vi "Red Pitaya Test.vi"(8 "Error In":errorcluster, 10 "Server port":u16=1002, 11 "Server address":string="192.168.1.100") -> (0 "Error Out":errorcluster)   [LabVIEW 2024]
uses:
  RP Command.ctl
  RP EEPROM Calibration.ctl
  RP Calibration.ctl
  RP Calibration 4ch.ctl
  RP Channel Calibration.ctl
  RP Filter 4ch.ctl
  RP Channel Filter.ctl
  RP Calibration 2ch.ctl
  RP Write Command TCP.vi
panel:
  out "Armed":bool
  in  "Trigger":bool
  in  "Arm":bool
  out "Numeric":dbl
  in  "length (rest)":i32
  in  "offset (0)":i32
  out "CH Calibration length":i32
  out "RP Calibration length":i32
  in  "New calibration format":bool=TRUE
  out "RP Calibration":T1
  out "RP EEPROM Calibration":T7 {"magic" format="%x"}
  in  "New connection":bool
  out "data out":string
  in  "Command payload":u64 format="%x"
  in  "Send Button":bool
  in  "Process Stop Button":bool
  in  "Command number":T8
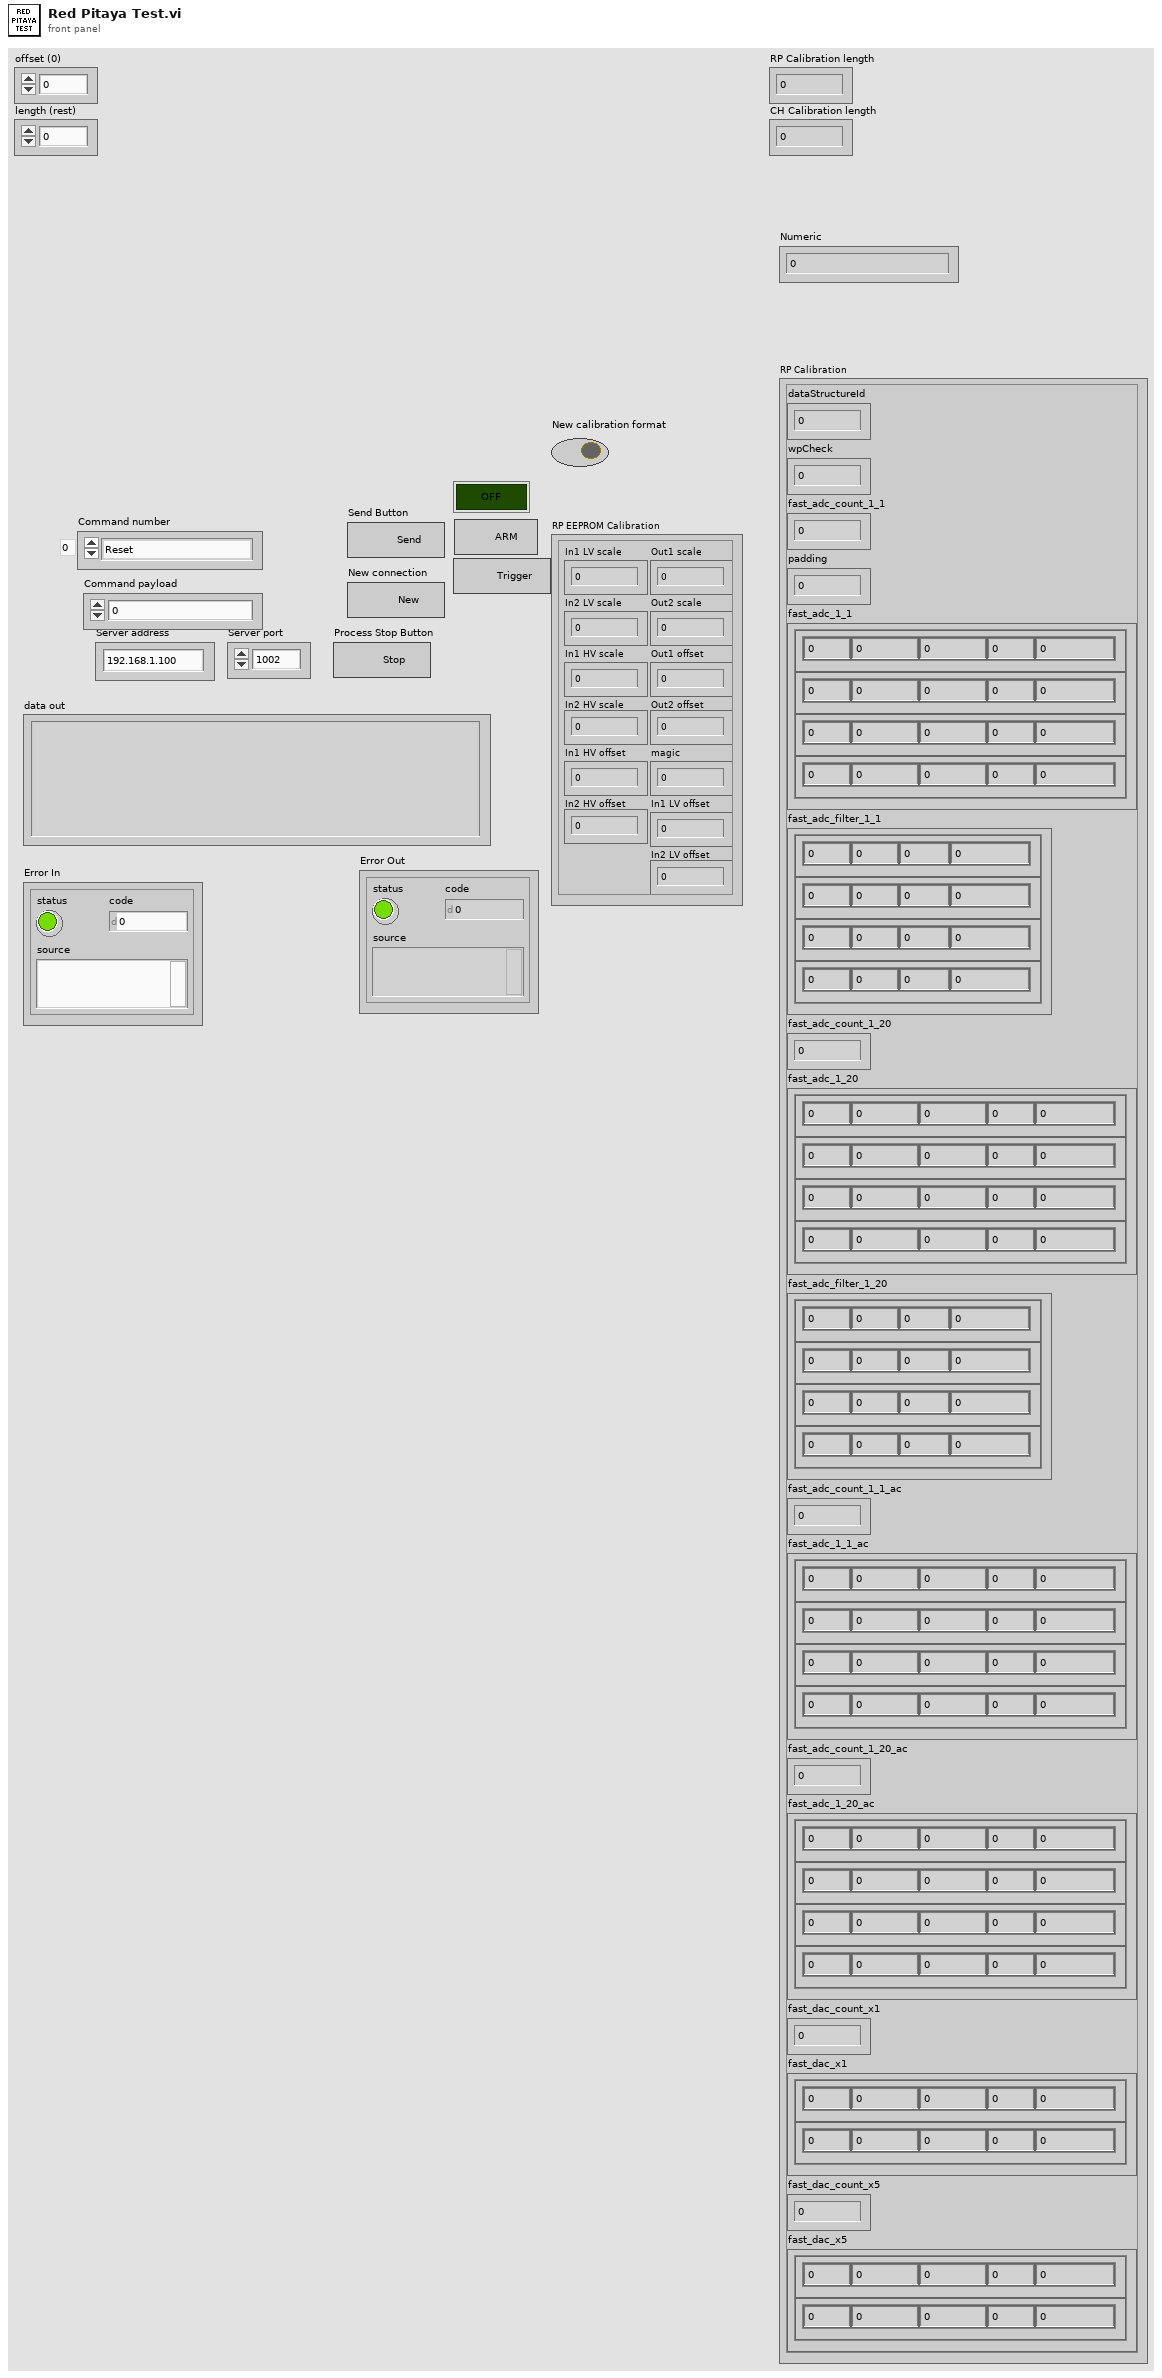
[diagram p1: front panel]
types:
  T1 = typedef "RP Calibration.ctl" = cluster{"dataStructureId":u8, "wpCheck":u8, "fast_adc_count_1_1":u16, "padding":u32, "fast_adc_1_1":T2, "fast_adc_filter_1_1":T4, "fast_adc_count_1_20":u64, "fast_adc_1_20":T2, "fast_adc_filter_1_20":T4, "fast_adc_count_1_1_ac":u64, "fast_adc_1_1_ac":T2, "fast_adc_count_1_20_ac":u64, "fast_adc_1_20_ac":T2, "fast_dac_count_x1":u64, "fast_dac_x1":T6, "fast_dac_count_x5":u64, "fast_dac_x5":T6}
  T2 = typedef "RP Calibration 4ch.ctl" = cluster{"ch_0":T3, "ch_1":T3, "ch_2":T3, "ch_3":T3}
  T3 = typedef "RP Channel Calibration.ctl" = cluster{"baseScale":sgl, "calibValue":u32, "offset":i32, "padding 2":i32, "gainCalc":dbl}
  T4 = typedef "RP Filter 4ch.ctl" = cluster{"ch_0":T5, "ch_1":T5, "ch_2":T5, "ch_3":T5}
  T5 = typedef "RP Channel Filter.ctl" = cluster{"aa":u32, "bb":u32, "pp":u32, "kk":u32}
  T6 = typedef "RP Calibration 2ch.ctl" = cluster{"ch_0":T3, "ch_1":T3}
  T7 = typedef "RP EEPROM Calibration.ctl" = cluster{"In1 LV scale":u32, "In2 LV scale":u32, "In1 HV scale":u32, "In2 HV scale":u32, "In1 HV offset":i32, "In2 HV offset":i32, "Out1 scale":u32, "Out2 scale":u32, "Out1 offset":i32, "Out2 offset":i32, "magic":u32, "In1 LV offset":i32, "In2 LV offset":i32}
  T8 = typedef "RP Command.ctl" = enum16{"Reset", "Read IDN", "Stop server", "Get status", "Get temperature", "Connect client", "Arm", "Software trigger", "Get whole buffer", "Get chunk", "System call", "Get config", "Set config", "Recieve data", "Recieve Calibartion", "Transmit data"}
  T9 = enum16{"big-endian, network order", "native, host order", "little-endian"}
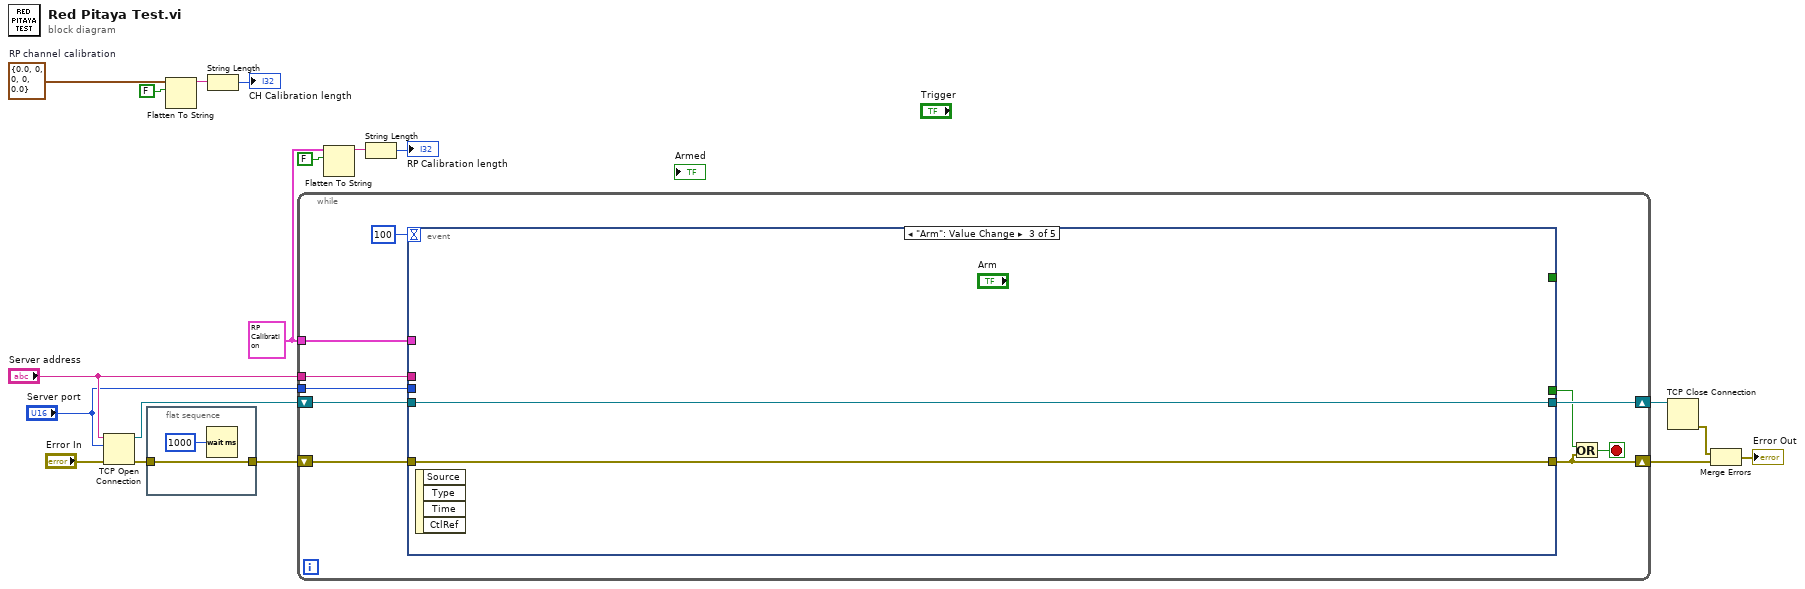
[diagram p0: block diagram]
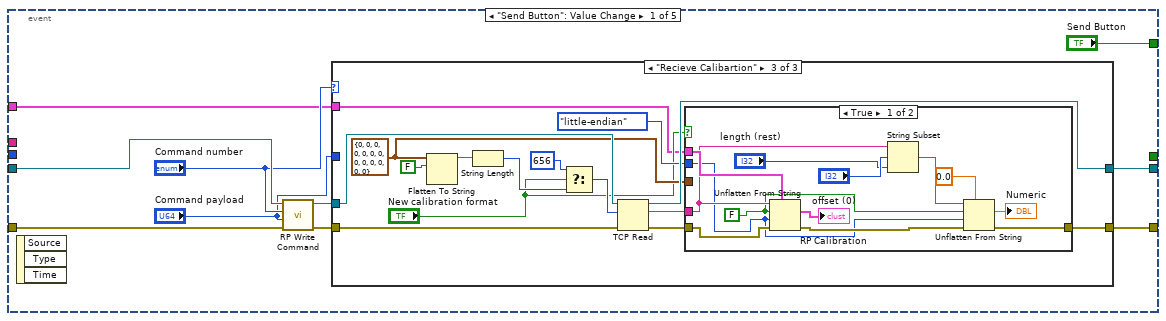
[diagram p2: hidden frame]
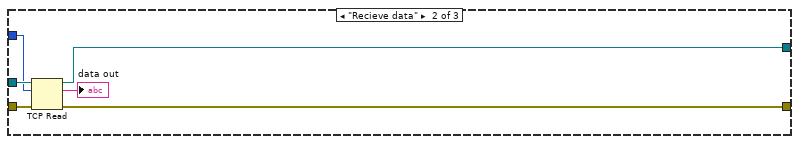
[diagram p4: hidden frame]
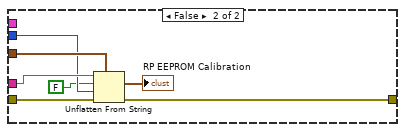
[diagram p5: hidden frame]
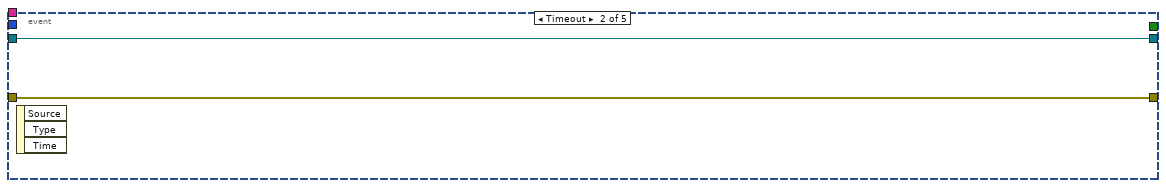
[diagram p6: hidden frame]
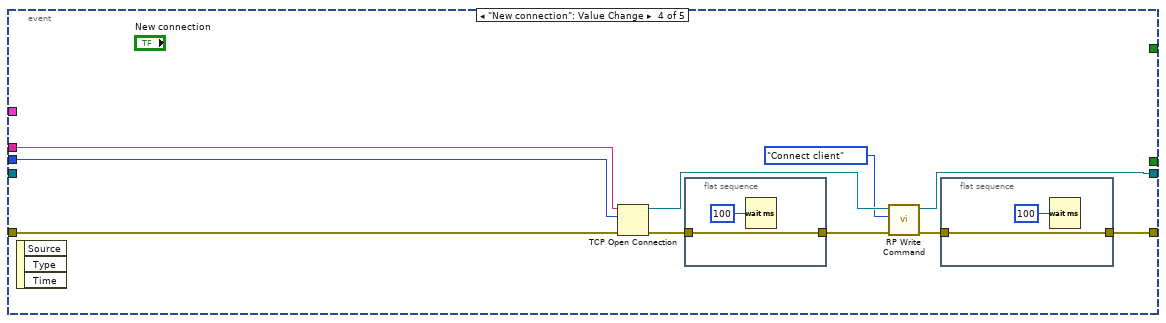
[diagram p7: hidden frame]
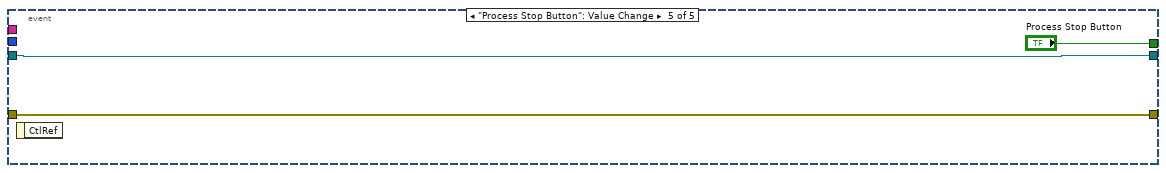
[diagram p8: hidden frame]
diagram:
  w1 = T1 {"dataStructureId"=0, "wpCheck"=0, "fast_adc_count_1_1"=0, "padding"=0, "fast_adc_1_1"={"ch_0"={"baseScale"=0.0, "calibValue"=0, "offset"=0, "padding 2"=0, "gainCalc"=0.0}, "ch_1"={"baseScale"=0.0, "calibValue"=0, "offset"=0, "padding 2"=0, "gainCalc"=0.0}, "ch_2"={"baseScale"=0.0, "calibValue"=0, "offset"=0, "padding 2"=0, "gainCalc"=0.0}, "ch_3"={"baseScale"=0.0, "calibValue"=0, "offset"=0, "padding 2"=0, "gainCalc"=0.0}}, "fast_adc_filter_1_1"={"ch_0"={"aa"=0, "bb"=0, "pp"=0, "kk"=0}, "ch_1"={"aa"=0, "bb"=0, "pp"=0, "kk"=0}, "ch_2"={"aa"=0, "bb"=0, "pp"=0, "kk"=0}, "ch_3"={"aa"=0, "bb"=0, "pp"=0, "kk"=0}}, "fast_adc_count_1_20"=0, "fast_adc_1_20"={"ch_0"={"baseScale"=0.0, "calibValue"=0, "offset"=0, "padding 2"=0, "gainCalc"=0.0}, "ch_1"={"baseScale"=0.0, "calibValue"=0, "offset"=0, "padding 2"=0, "gainCalc"=0.0}, "ch_2"={"baseScale"=0.0, "calibValue"=0, "offset"=0, "padding 2"=0, "gainCalc"=0.0}, "ch_3"={"baseScale"=0.0, "calibValue"=0, "offset"=0, "padding 2"=0, "gainCalc"=0.0}}, "fast_adc_filter_1_20"={"ch_0"={"aa"=0, "bb"=0, "pp"=0, "kk"=0}, "ch_1"={"aa"=0, "bb"=0, "pp"=0, "kk"=0}, "ch_2"={"aa"=0, "bb"=0, "pp"=0, "kk"=0}, "ch_3"={"aa"=0, "bb"=0, "pp"=0, "kk"=0}}, "fast_adc_count_1_1_ac"=0, "fast_adc_1_1_ac"={"ch_0"={"baseScale"=0.0, "calibValue"=0, "offset"=0, "padding 2"=0, "gainCalc"=0.0}, "ch_1"={"baseScale"=0.0, "calibValue"=0, "offset"=0, "padding 2"=0, "gainCalc"=0.0}, "ch_2"={"baseScale"=0.0, "calibValue"=0, "offset"=0, "padding 2"=0, "gainCalc"=0.0}, "ch_3"={"baseScale"=0.0, "calibValue"=0, "offset"=0, "padding 2"=0, "gainCalc"=0.0}}, "fast_adc_count_1_20_ac"=0, "fast_adc_1_20_ac"={"ch_0"={"baseScale"=0.0, "calibValue"=0, "offset"=0, "padding 2"=0, "gainCalc"=0.0}, "ch_1"={"baseScale"=0.0, "calibValue"=0, "offset"=0, "padding 2"=0, "gainCalc"=0.0}, "ch_2"={"baseScale"=0.0, "calibValue"=0, "offset"=0, "padding 2"=0, "gainCalc"=0.0}, "ch_3"={"baseScale"=0.0, "calibValue"=0, "offset"=0, "padding 2"=0, "gainCalc"=0.0}}, "fast_dac_count_x1"=0, "fast_dac_x1"={"ch_0"={"baseScale"=0.0, "calibValue"=0, "offset"=0, "padding 2"=0, "gainCalc"=0.0}, "ch_1"={"baseScale"=0.0, "calibValue"=0, "offset"=0, "padding 2"=0, "gainCalc"=0.0}}, "fast_dac_count_x5"=0, "fast_dac_x5"={"ch_0"={"baseScale"=0.0, "calibValue"=0, "offset"=0, "padding 2"=0, "gainCalc"=0.0}, "ch_1"={"baseScale"=0.0, "calibValue"=0, "offset"=0, "padding 2"=0, "gainCalc"=0.0}}} ("RP Calibration")
  w4 = T3 {"baseScale"=0.0, "calibValue"=0, "offset"=0, "padding 2"=0, "gainCalc"=0.0}  # RP channel calibration
  n1 = TCP Open Connection(address="Server address", remote port or service name="Server port", error in (no error)="Error In") -> (connection ID=w14:refnum<k5>, error out=w13:errorcluster)  [unwired: 2 in]
  n2 = flat-sequence {
    tunnel: w13 -> [w19]
    tunnel: [w19] -> w12
    frame #0 {
      n3 = Wait (ms)(milliseconds to wait=u32 1000) -> ()  [unwired: 1 out]
    }
  }
  n4 = Flatten To String(anything=w4, prepend array or string size? (T)=FALSE) -> (data string=w2:string)  [unwired: 2 in, 2 out]
  n5 = String Length(string=w2) -> (length=→"CH Calibration length":i32)
  n6 = while {
    shift-right: [w30] -> w16
    shift-left: w14 -> [w29]
    shift-right: [w25] -> w15
    shift-left: w12 -> [w28]
    tunnel: "Server address" -> [w23]
    tunnel: "Server port" -> [w22]
    tunnel: w1 -> [w21]
    stop <- w26 stop-if-true
    n7 = event shown="[2] \"Arm\": Value Change" {
      selector: _ -> [_ _ _ _ _]
      dyn-events: _ -> [_ _ _ _ _]
      timeout: 100 -> [_ _ _ _ _]
      tunnel: [w33 w85 w86 w88 w102] -> w30
      tunnel: [w32 w84 w87 w89 w103] -> w25
      tunnel: w29 -> [w40 w85 w86 _ w102]
      tunnel: w28 -> [w39 w84 w87 w97 w103]
      tunnel: [_ _ _ _ "Process Stop Button"] -> w27
      tunnel: ["Send Button" _ _ _ _] -> _
      tunnel: w23 -> [_ _ _ w96 _]
      tunnel: w22 -> [_ _ _ w95 _]
      tunnel: w21 -> [w31 _ _ _ _]
      event "Send Button": Value Change {
        n8 = event-data() -> ()  [unwired: 1 in, 3 out]
        n9 = call-poly "RP Write Command.vi"("Error In"=w39, "Command payload"="Command payload", "Command number"="Command number", "connection ID"=w40) -> ("Error Out"=w37:errorcluster, "connection ID out"=w34:refnum<k5>)  [unwired: 4 in, 2 out]
        n10 = case shown="\"Recieve Calibartion\"" "Command number" {
          tunnel: w37 -> [w41 w48 w63]
          tunnel: "Command payload" -> [_ w46 _]
          tunnel: w34 -> [w42 w47 w62]
          tunnel: [w42 w45 w61] -> w33
          tunnel: [w41 w44 w55] -> w32
          tunnel: w31 -> [_ _ w49]
          frame "Reset", Default {
          }
          frame "Recieve data" {
            n11 = TCP Read(connection ID=w47, bytes to read=w46, error in (no error)=w48) -> (connection ID out=w45:refnum<k5>, data out=→"data out":string, error out=w44:errorcluster)  [unwired: 2 in]
          }
          frame "Recieve Calibartion" {
            w57 = T7 {"In1 LV scale"=0, "In2 LV scale"=0, "In1 HV scale"=0, "In2 HV scale"=0, "In1 HV offset"=0, "In2 HV offset"=0, "Out1 scale"=0, "Out2 scale"=0, "Out1 offset"=0, "Out2 offset"=0, "magic"=0, "In1 LV offset"=0, "In2 LV offset"=0} ("RP EEPROM Calibration")
            n12 = Flatten To String(anything=w57, prepend array or string size? (T)=FALSE) -> (data string=w59:string)  [unwired: 2 in, 2 out]
            n13 = String Length(string=w59) -> (length=w52:i32)
            n14 = Select(t=656, s="New calibration format", f=w52) -> (s? t:f=w51:i32)
            n15 = TCP Read(connection ID=w62, bytes to read=w51, error in (no error)=w63) -> (connection ID out=w61:refnum<k5>, data out=w58:string, error out=w56:errorcluster)  [unwired: 2 in]
            n16 = case shown="True" "New calibration format" {
              tunnel: w58 -> [w73 w83]
              tunnel: w57 -> [_ w82]
              tunnel: w56 -> [w76 w80]
              tunnel: [w68 w79] -> w55
              tunnel: T9."little-endian" ("byte order (0:big-endian, network order)") -> [w64 w78]
              tunnel: w49 -> [w74 _]
              frame True {
                w65 = FALSE ("data includes array or string size? (T)")
                n17 = Unflatten From String(type=w74, binary string=w73, data includes array or string size? (T)=w65, byte order (0:big-endian, network order)=w64, error in (no error)=w76) -> (value=→"RP Calibration":T1, error out=w69:errorcluster)  [unwired: 1 out]
                n18 = String Subset(string=w73, offset (0)="offset (0)", length (rest)="length (rest)") -> (substring=w66:string)
                n19 = Unflatten From String(type=0.0 ("Numeric"), binary string=w66, data includes array or string size? (T)=w65, byte order (0:big-endian, network order)=w64, error in (no error)=w69) -> (value=→"Numeric":dbl, error out=w68:errorcluster)  [unwired: 1 out]
              }
              frame False {
                n20 = Unflatten From String(type=w82, binary string=w83, data includes array or string size? (T)=FALSE, byte order (0:big-endian, network order)=w78, error in (no error)=w80) -> (value=→"RP EEPROM Calibration":T7, error out=w79:errorcluster)  [unwired: 1 out]
              }
            }
          }
        }
      }
      event Timeout {
        n21 = event-data() -> ()  [unwired: 1 in, 3 out]
      }
      event "Arm": Value Change {
        n22 = event-data() -> ()  [unwired: 1 in, 4 out]
      }
      event "New connection": Value Change {
        n23 = event-data() -> ()  [unwired: 1 in, 3 out]
        n24 = TCP Open Connection(address=w96, remote port or service name=w95, error in (no error)=w97) -> (connection ID=w92:refnum<k5>, error out=w94:errorcluster)  [unwired: 2 in]
        n25 = flat-sequence {
          tunnel: w94 -> [w100]
          tunnel: [w100] -> w93
          frame #0 {
            n26 = Wait (ms)(milliseconds to wait=u32 100) -> ()  [unwired: 1 out]
          }
        }
        n27 = call-poly "RP Write Command.vi"("Error In"=w93, "Command number"=RP_Command."Connect client", "connection ID"=w92) -> ("Error Out"=w90:errorcluster, "connection ID out"=w88:refnum<k5>)  [unwired: 5 in, 2 out]
        n28 = flat-sequence {
          tunnel: w90 -> [w98]
          tunnel: [w98] -> w89
          frame #0 {
            n29 = Wait (ms)(milliseconds to wait=u32 100) -> ()  [unwired: 1 out]
          }
        }
      }
      event "Process Stop Button": Value Change {
        n30 = event-data() -> ()  [unwired: 1 in, 1 out]
      }
    }
    n31 = Or(x=w27, y=w25) -> (x .or. y?=w26:bool)
  }
  n32 = Flatten To String(anything=w1, prepend array or string size? (T)=FALSE) -> (data string=w8:string)  [unwired: 2 in, 2 out]
  n33 = String Length(string=w8) -> (length=→"RP Calibration length":i32)
  n34 = TCP Close Connection(connection ID=w16) -> (error out=w18:errorcluster)  [unwired: 2 in, 1 out]
  n35 = Merge Errors(w18, w15) -> (→"Error Out":errorcluster)
